vi "Graph3D.vi"(0 "Experiment3D in":refnum<class "Experiment3D.lvclass">, 5 "error in (no error)":errorcluster) -> (14 "Experiment3D out":refnum<class "Experiment3D.lvclass">, 15 "Finish?":bool, 16 "X":dbl[](array[numeric]), 17 "Y":dbl[](array[numeric]), 18 "Z matrix":dbl[][](array[numeric]), 19 "error out":errorcluster)   [LabVIEW 2014, in "Experiment3D.lvclass"]
uses:
  Experiment3D.lvclass
  Measurement/Measurement3D/Measurement3D.lvclass
  Data/Data3D/Data3D.lvclass
  <vilib>/Math Plots/3D Math Plots/3D Surface/3D Surface Datatype/3D Surface Datatype.lvclass
  <vilib>/Math Plots/3D Math Plots/3D Surface/3D Surface Datatype/Public/Plot Helper (Vector).vi
  <vilib>/Math Plots/3D Math Plots/3D Surface/3D Surface XCtrl/3D Surface.xctl
panel:
  out "3D Surface":refnum<class "3D Plot Datatype.lvclass">[](xcontrol)
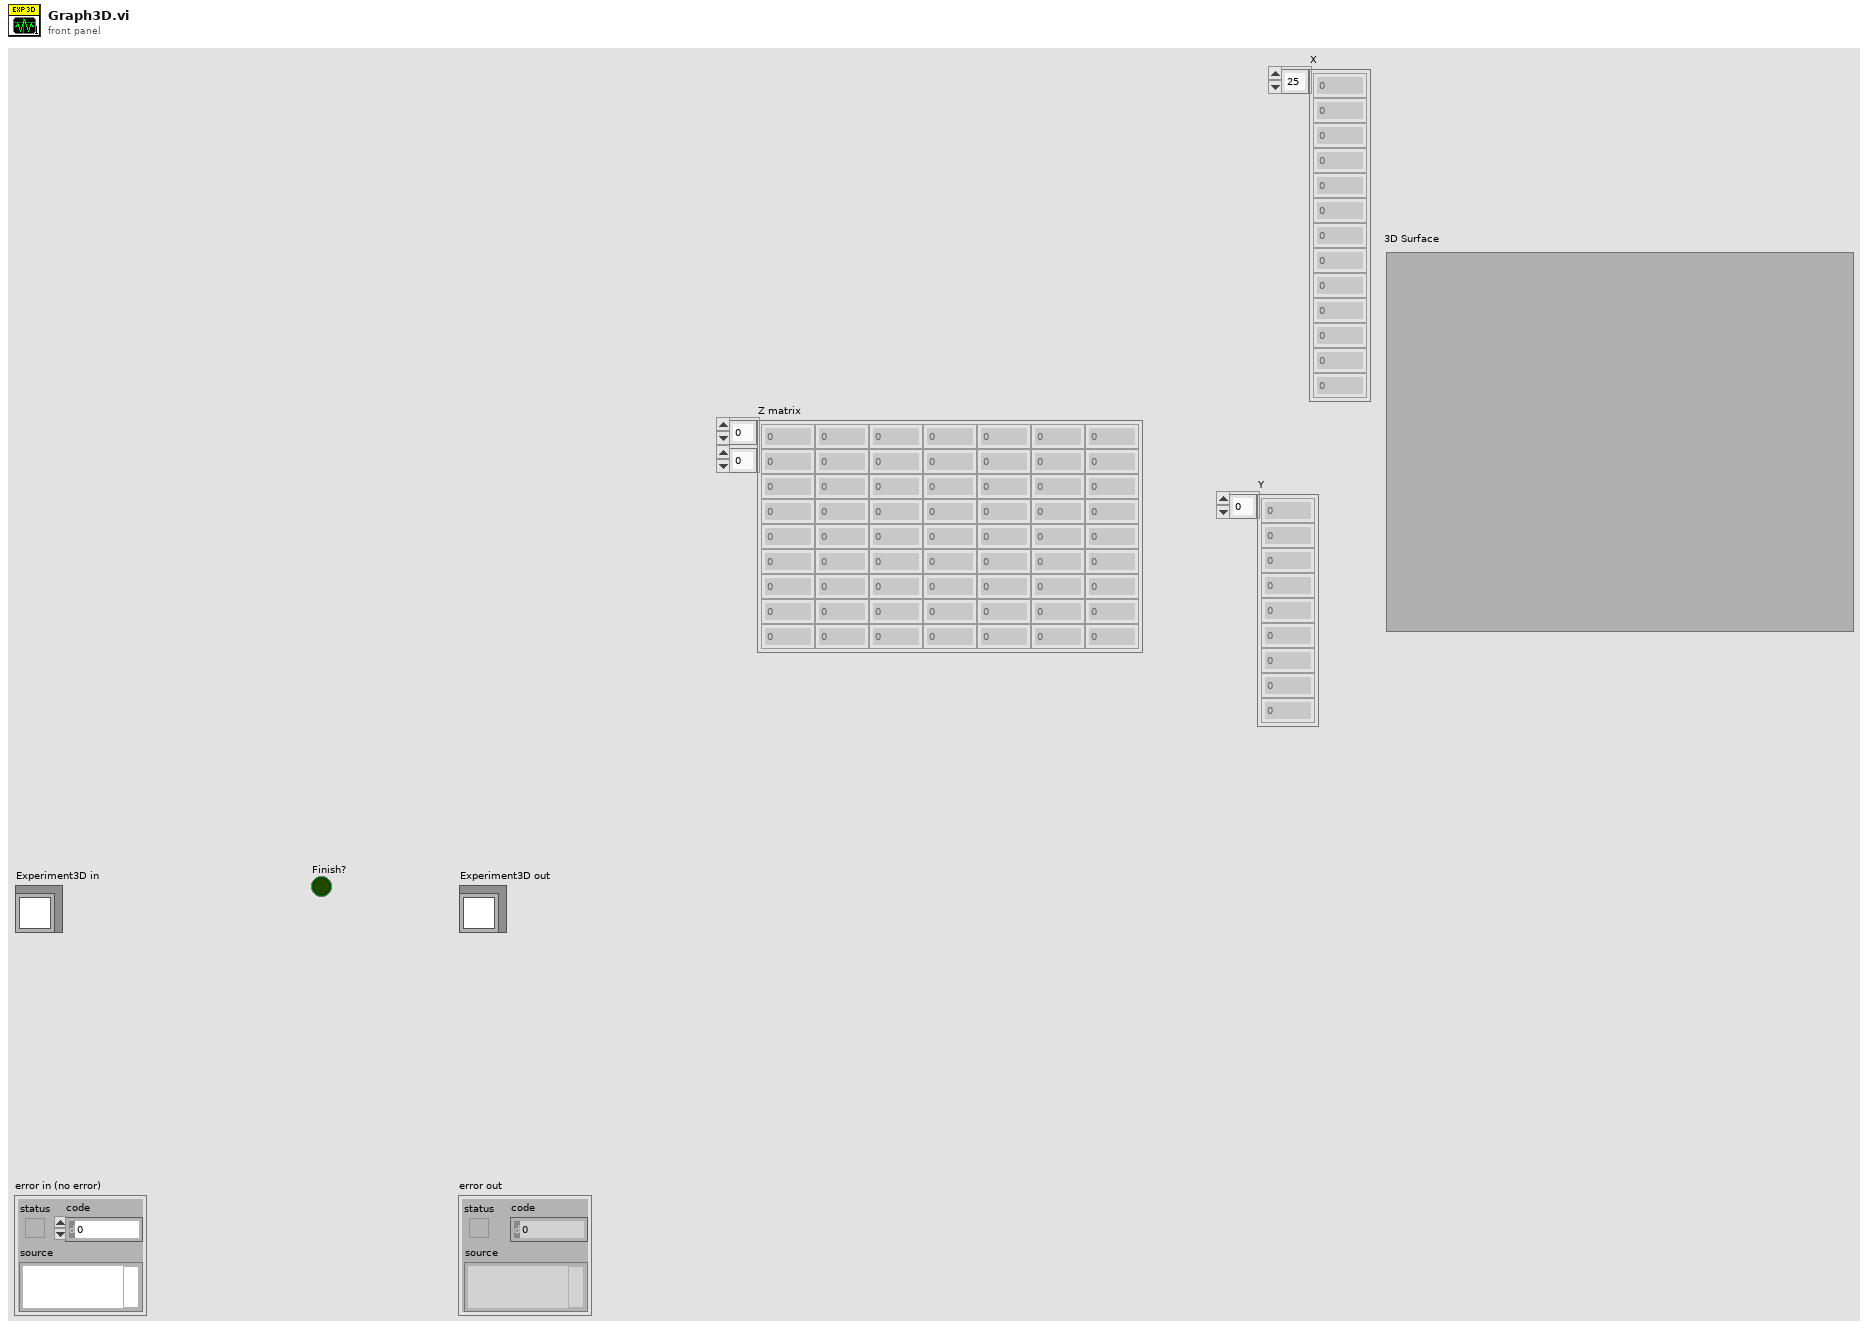
[diagram p1: front panel]
types:
  T1 = cluster{"Init":dbl, "Step":dbl, "Max":dbl, "Current Value":dbl, "Current Index":dbl, "Sweep Outer":dbl[]}
  T2 = cluster{"Init":dbl, "Step":dbl, "Max":dbl, "Current Value":dbl, "Current Index":dbl, "Sweep Inner":dbl[]}
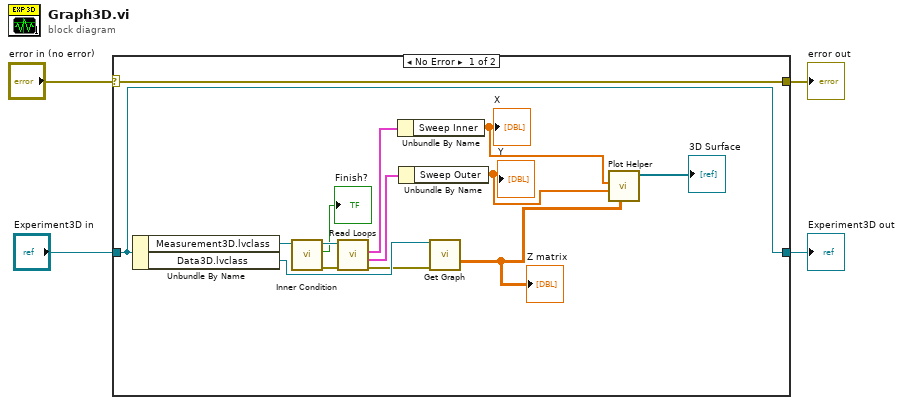
[diagram p0: block diagram]
diagram:
  n1 = case shown="No Error" "error in (no error)" {
    selector: "error in (no error)" -> [w18 w20]
    tunnel: [w18 w20] -> w3
    tunnel: [w17 w19] -> w1
    tunnel: "Experiment3D in" -> [w17 w19]
    frame No Error {
      n2 = Unbundle By Name(w17) -> ("Measurement3D.lvclass"=w16:refnum<class "Measurement3D.lvclass">, "Data3D.lvclass"=w15:refnum<class "Data3D.lvclass">)
      n3 = call "Inner Condition.vi"("Measurement3D in"=w16) -> ("error out"=w11:errorcluster, "Finish?"=→"Finish?":bool, "Measurement3D out"=w12:refnum<class "Measurement3D.lvclass">)  [unwired: 8 in]
      n4 = call "Read Loops.vi"("error in (no error)"=w11, "Measurement3D in"=w12) -> ("error out"=w10:errorcluster, "Outer Loop"=w13:T1, "Inner Loop"=w14:T2)  [unwired: 6 in, 1 out]
      n5 = Unbundle By Name(w14) -> ("Sweep Inner"=w6:dbl[])
      "X" <- w6
      n6 = Unbundle By Name(w13) -> ("Sweep Outer"=w5:dbl[])
      "Y" <- w5
      n7 = call "Get Graph.vi"("Data3D in"=w15, "error in (no error)"=w10) -> ("Z matrix"=w7:dbl[][])  [unwired: 9 in, 4 out]
      "Z matrix" <- w7
      n8 = call-poly <vilib>:"Plot Helper.vi"("z matrix"=w7, "y vector"=w5, "x vector"=w6) -> ("3D Plot lvclass Array out"=→"3D Surface":refnum<class "3D Plot Datatype.lvclass">[])  [unwired: 3 in, 5 out]
    }
    frame Error {
    }
  }
  "error out" <- w3
  "Experiment3D out" <- w1
